vi "Implode String.vi"(7 "Delimiter (,)":string=",", 11 "Array":string[](array[string])) -> (3 "String":string)   [LabVIEW 2020, in "Negentropic IDE.lvlib"]
uses:
  Negentropic IDE.lvlib
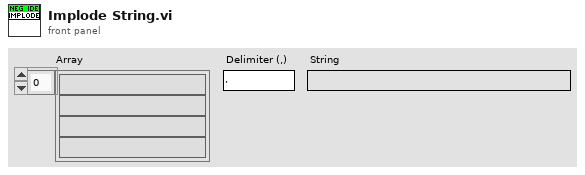
[diagram p1: front panel]
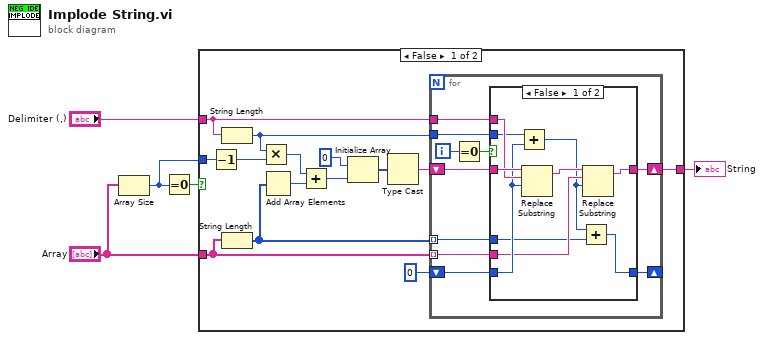
[diagram p0: block diagram]
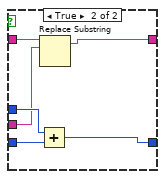
[diagram p2: hidden frame]
diagram:
  n1 = Array Size(array="Array") -> (size(s)=w3:i32)
  n2 = Equal To 0?(x=w3) -> (x = 0?=w5:bool)
  n3 = case shown="False" w5 {
    tunnel: "Array" -> [w12 _]
    tunnel: w3 -> [w19 _]
    tunnel: "Delimiter (,)" -> [w8 _]
    tunnel: [w7 _] -> w1
    frame False {
      n4 = Decrement(x=w19) -> (x-1=w18:i32)
      n5 = String Length(string=w8) -> (length=w9:i32)
      n6 = String Length(string=w12) -> (length=w11:i32[])
      n7 = Multiply(x=w9, y=w18) -> (x*y=w16:i32)
      n8 = Add Array Elements(numeric array=w11) -> (sum=w17:i32)
      n9 = Add(x=w16, y=w17) -> (x+y=w15:i32)
      n10 = Initialize Array(u8 0 ("element"), w15) -> (w13:u8[])
      n11 = Type Cast(x=w13) -> (*(type *) &x=w10:string)  [unwired: 1 in]
      n12 = for {
        tunnel: w12 -> [w23] mode=indexing
        tunnel: w11 -> [w24] mode=indexing
        shift-right: [w20] -> w7
        shift-left: w10 -> [w25]
        tunnel: w9 -> [w27]
        tunnel: w8 -> [w26]
        shift-right: [w21] -> _
        shift-left: 0 ("element") -> [w22]
        i -> [w29]
        n13 = Equal To 0?(x=w29) -> (x = 0?=w28:bool)
        n14 = case shown="False" w28 {
          tunnel: w27 -> [w37 _]
          tunnel: w26 -> [w38 _]
          tunnel: w25 -> [w39 w45]
          tunnel: w24 -> [w33 w41]
          tunnel: w23 -> [w34 w40]
          tunnel: w22 -> [w36 w43]
          tunnel: [w31 w42] -> w21
          tunnel: [w30 w44] -> w20
          frame False {
            n15 = Add(x=w37, y=w36) -> (x+y=w32:i32)
            n16 = Replace Substring(3:w36, 4:w38, 5:w39) -> (1:w35:string)  [unwired: 1 in, 1 out]
            n17 = Add(x=w32, y=w33) -> (x+y=w31:i32)
            n18 = Replace Substring(3:w32, 4:w34, 5:w35) -> (1:w30:string)  [unwired: 1 in, 1 out]
          }
          frame True {
            n19 = Add(x=w41, y=w43) -> (x+y=w42:i32)
            n20 = Replace Substring(4:w40, 5:w45) -> (1:w44:string)  [unwired: 2 in, 1 out]
          }
        }
      }
    }
    frame True {
    }
  }
  "String" <- w1
